vi "Wind_Turbine.vi"() -> (5 "Plug in titles":string[](array[string]), 7 "Plug in values":string[](array[string]))   [LabVIEW 2010]
uses:
  Globals/Meas_global.vi
  Globals/Plug_in_data_global.vi
  Globals/LDA_meas_global_1.vi
  Plug in sub vis/Wind_Turbine_Global.vi
  <vilib>/Analysis/NI_AALBase.lvlib
  <vilib>/Analysis/NI_AALPro.lvlib
panel:
  out "Angle 3":dbl format="%#_3g"
  out "Angle 2":dbl format="%#_3g"
  out "Angle 1":dbl format="%#_3g"
  out "L Status Phase lock index":i32
  out "Laser Status Index":i32
  out "Waveform Graph 3":dbl[](graph)
  out "Laser Phase lock index":i32
  out "Laser Disp Index":i32
  out "Av Variance 3":dbl
  out "Av Variance 2":dbl
  out "Av Variance 1":dbl
  out "slope 3":dbl format="%#_3g"
  out "slope 2":dbl format="%#_3g"
  out "Variance Blade 3":dbl[](graph)
  out "Variance Blade 2":dbl[](graph)
  out "Mean Blade 3":dbl[](graph)
  out "Mean Blade 2":dbl[](graph)
  out "Variance Blade 1":dbl[](graph)
  out "Av Disp 3":dbl
  out "Av Disp 2":dbl
  out "Av Disp 1":dbl
  out "slope 1":dbl format="%#_3g"
  in  "End Cut Deg":dbl
  in  "Start Cut Deg":dbl
  out "Waveform Graph 2":i16[](graph)
  out "Mean Blade 1":dbl[](graph)
  out "Array":i32[](array[numeric])
  in  "Angular Step":dbl=0.1
  in  "Turbine to Phase Lock to":u16(ring) items=["RV (WT1)"]
  in  "Change Dem Voltages?":bool
  out "All WTs":dbl[][](array[numeric]) format="%#.2g"
  out "WT trace index":i32[](array[numeric])
  in  "precision":string
  in  "Add Phase data to results file":bool
  in  "Separation Character":string="\t"
  in  "Output Directory":path
  in  "Save Phase averaged Profiles":bool
  out "LDA Chs":i32[](array[numeric])
  out "WT Stalled?":bool
  out "Pulse No":i32
  out "Last index":i32
  out "subarray":bool[](array[boolean])
  out "Index":i32[](array[numeric])
  out "Pulses per Rev":i32
  out "Av samples per pulse":i32
  out "Threshold":dbl
  in  "Channel to Phase lock":i32[](listbox)
  out "Last Block No of Revs":i32
  out "Hub RPM":dbl
  out "Generator trace":cluster{dbl, dbl, dbl[]}(graph)
  out "Hot wire trace":cluster{dbl, dbl, dbl[][]}(graph)
  out "Number of Revs":i32
  # "Mean RPM      SD RPM           Max-Min"
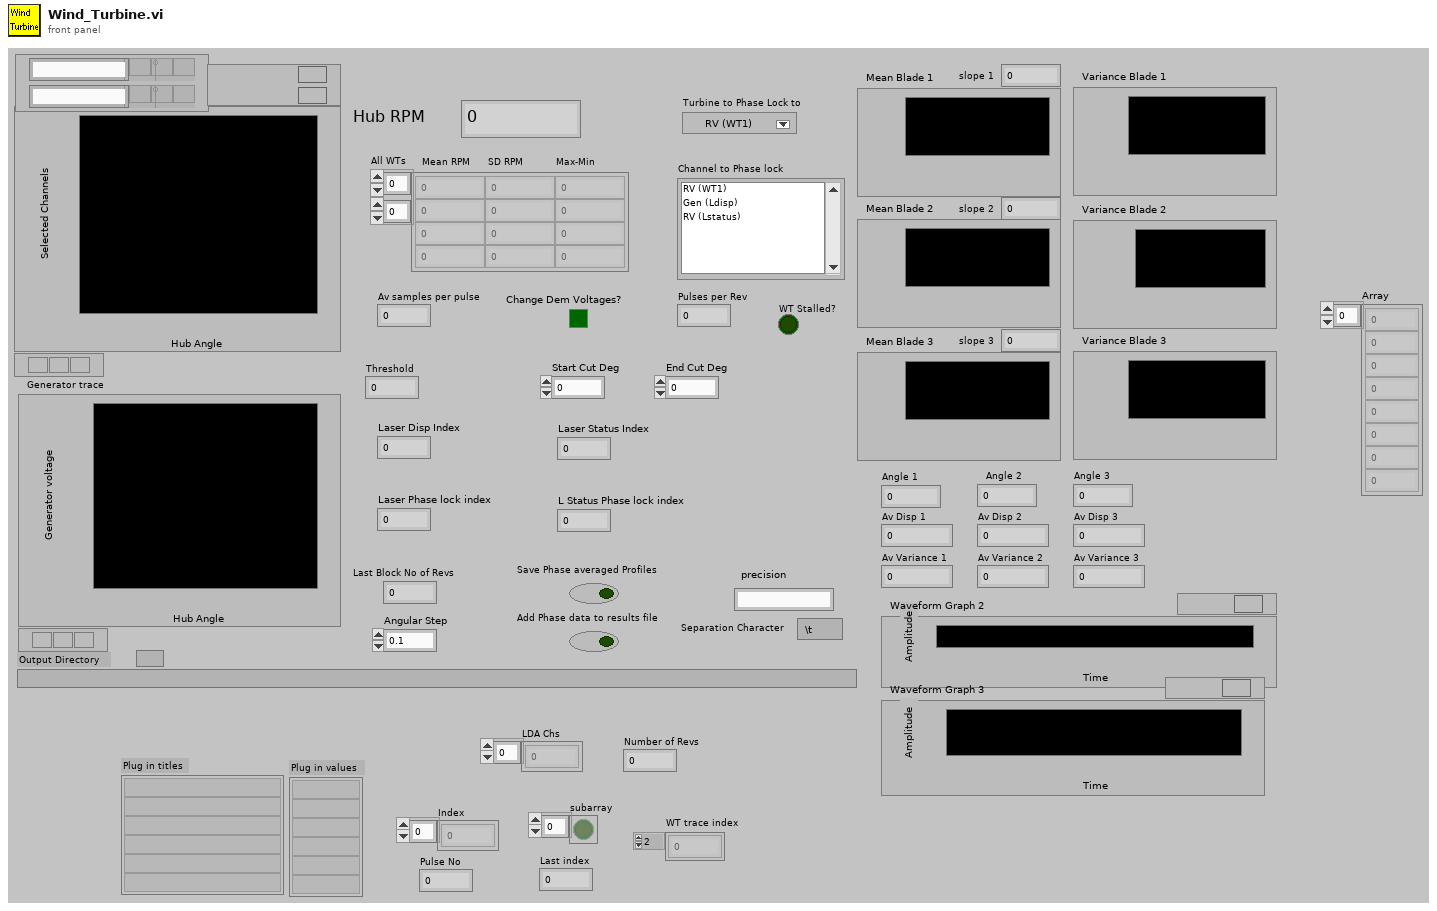
[diagram p1: front panel]
types:
  T1 = typedef "Analysis_info_cluster.ctl" = cluster{"Colour":u32, "Inst type":T2, "Inst name":string, "Symbol":string, "Code name":string, "Extra Info":string, "Inst Array":T3, "Index":i32, "Voltage Index":i32, "Extra Titles":string[], "Extra Values":string[]}
  T2 = typedef "Inst_type.ctl" = enum16{"Propeller anemometer", "Raw voltage", "Pressure Transducer", "Pitot-static tube", "Preston tube", "Hot wire", "Cross wire 1", "Cross wire 2", "Generic Linear", "Generic Polynomial", "Generic BackPoly", "Fast FID", "Thermocouple", "Cold wire", "Pulsed Wire", "LDA Vel", "LDA Tran time", "LDA Arr time"}
  T3 = typedef "Instrument_Array.ctl" = enum16{"PWA", "LDA", "Analogue"}
  T4 = typedef "Post_Process.ctl" = enum16{"Take New Data", "Post Process Raw Data File"}
  T5 = cluster{"Name":string, "X":dbl, "Y":dbl, "Z":dbl}[]
  T6 = cluster{"Name":string, "X":dbl, "Y":dbl, "Z":dbl}
  T7 = cluster{"[0]":bool, "[1]":bool, "[2]":bool, "[3]":bool}
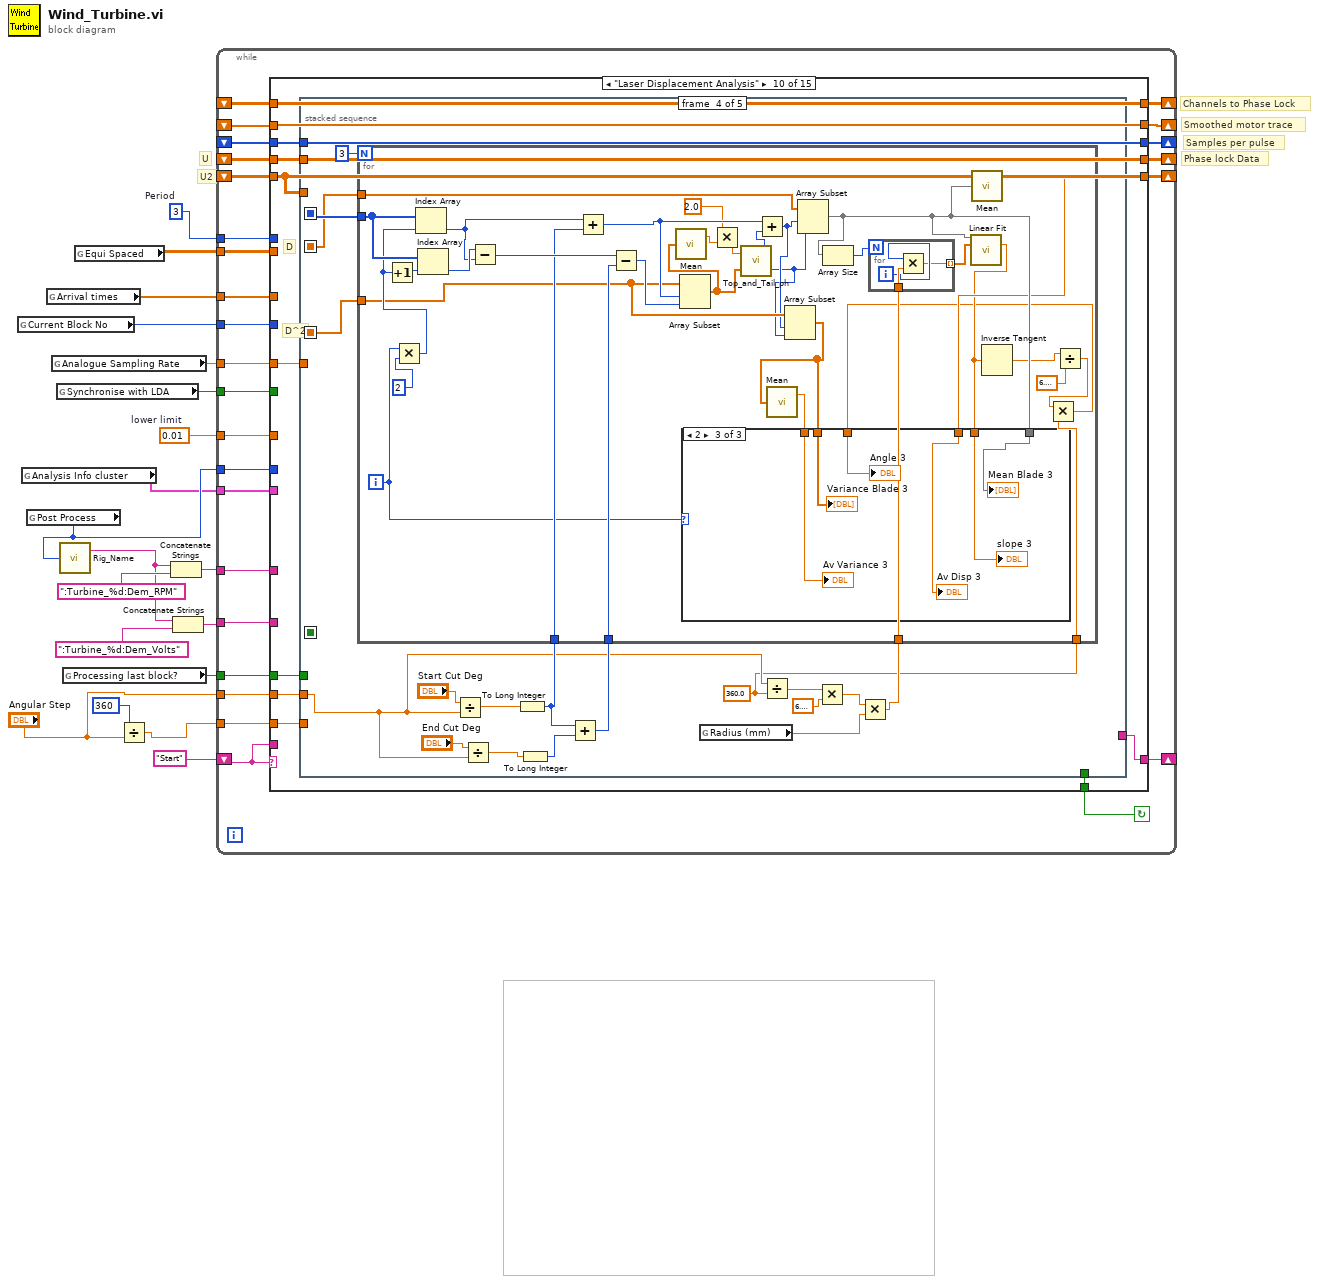
[diagram p0: block diagram]
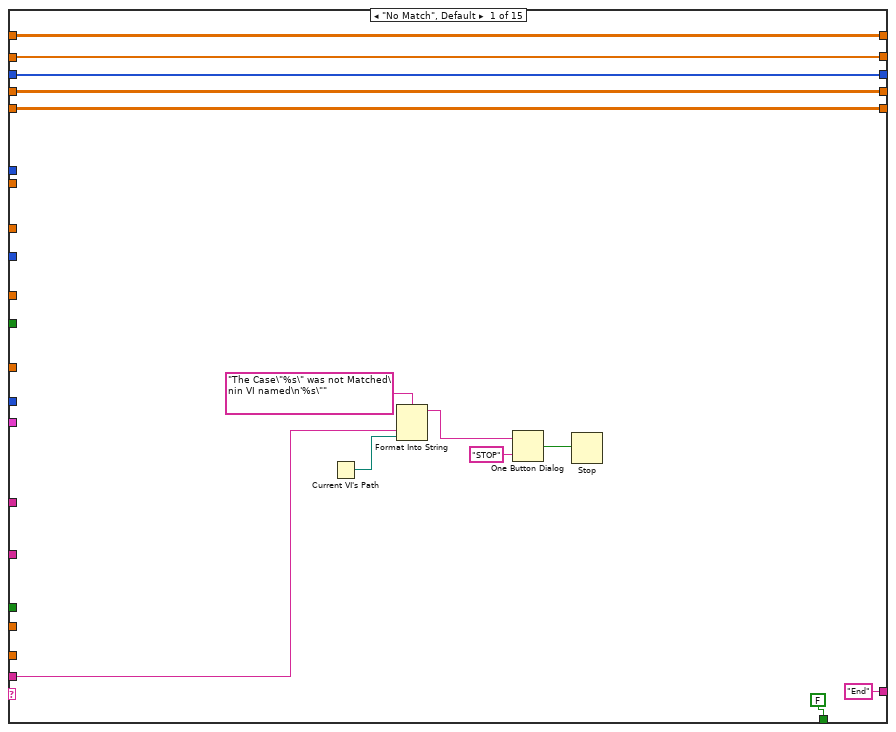
[diagram p2: hidden frame]
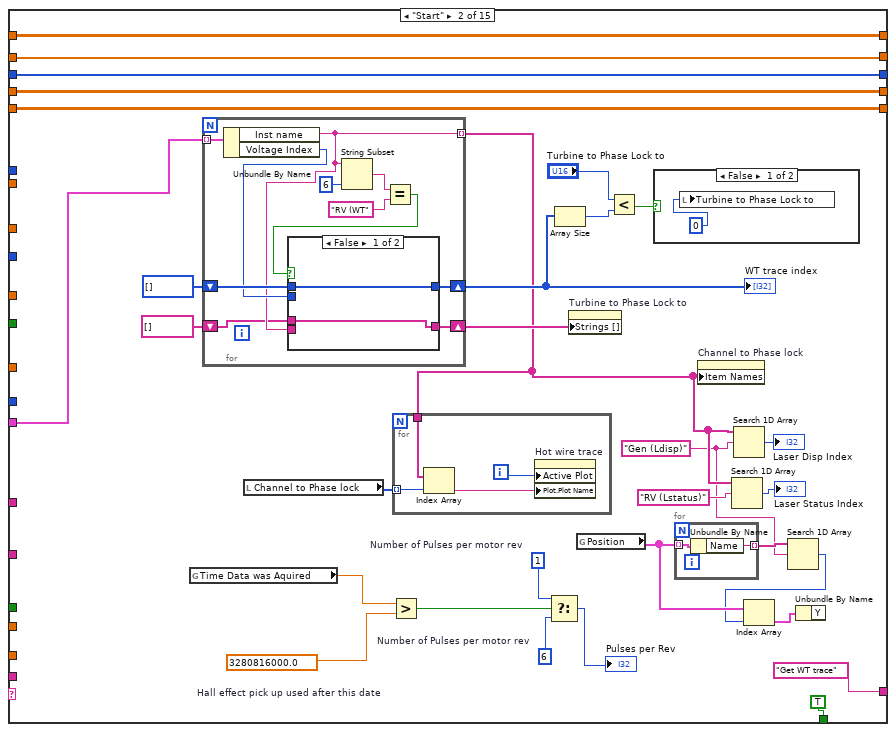
[diagram p3: hidden frame]
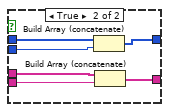
[diagram p5: hidden frame]
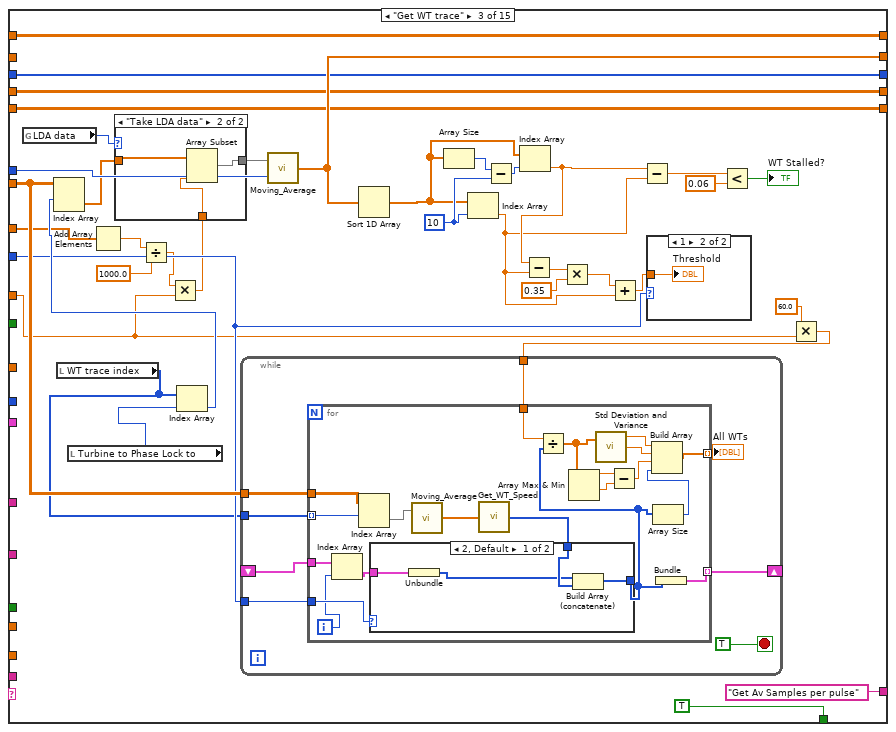
[diagram p6: hidden frame]
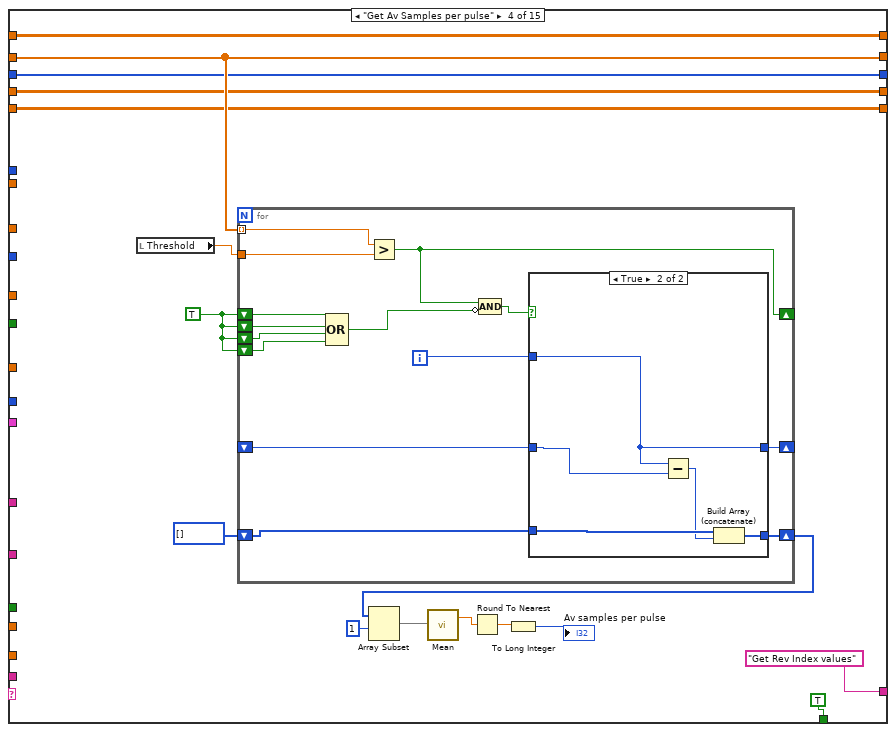
[diagram p10: hidden frame]
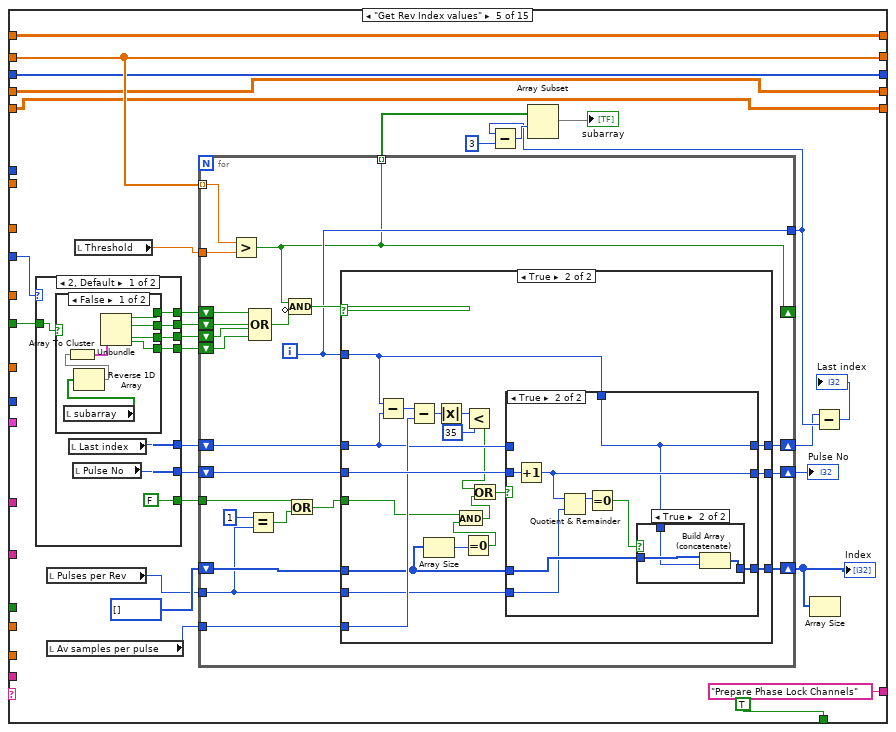
[diagram p12: hidden frame]
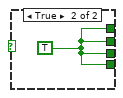
[diagram p13: hidden frame]
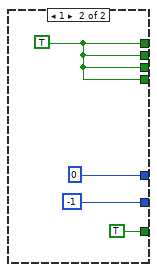
[diagram p14: hidden frame]
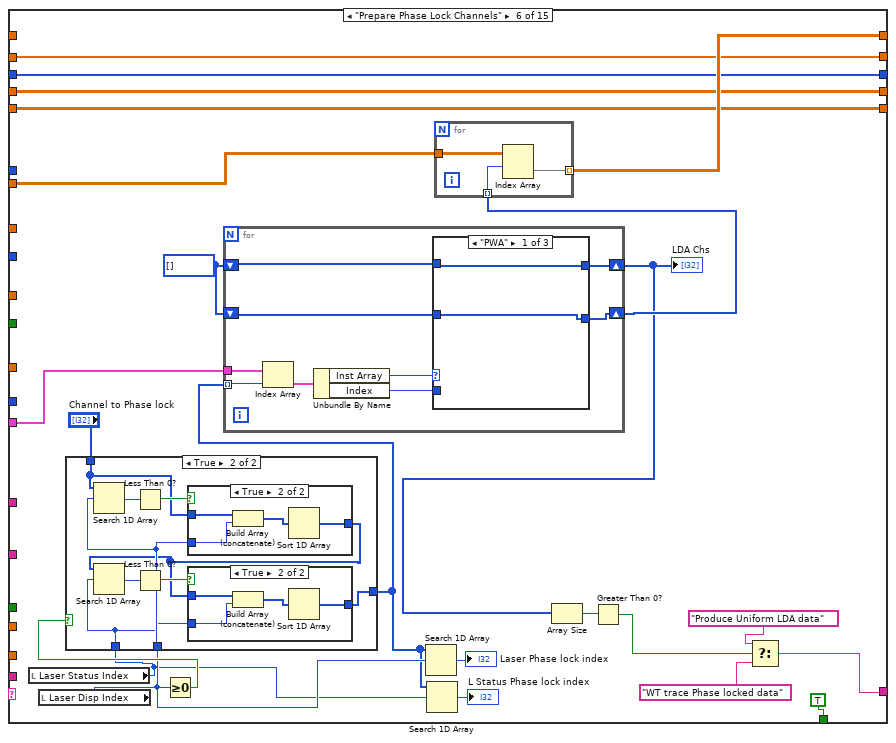
[diagram p18: hidden frame]
diagram:
  w16 = 3  # Period
  w17 = 0.01  # lower limit
  # "U"
  # "U2"
  # "Channels to Phase Lock"
  # "Phase lock Data"
  # "Samples per pulse"
  # "Smoothed motor trace"
  n1 = global read "Meas_global.vi" "Current Block No"() -> (w19:i32)
  n2 = global read "Meas_global.vi" "Analysis Info cluster"() -> (w8:T1[])
  n3 = global read "Meas_global.vi" "Post Process"() -> (w15:T4)
  n4 = global read "LDA_meas_global_1.vi" "Arrival times"() -> (w2:dbl[])
  n5 = global read "Meas_global.vi" "Analogue Sampling Rate"() -> (w18:dbl)
  n6 = global read "Meas_global.vi" "Synchronise with LDA"() -> (w9:bool)
  n7 = call "Rig_Name.vi"("Post Process"=w15) -> ("Rig Setup before dash"=w11:string)  [unwired: 1 out]
  n8 = global read "Meas_global.vi" "Processing last block?"() -> (w6:bool)
  n9 = global read "Plug_in_data_global.vi" "Equi Spaced"() -> (w5:dbl[][])
  n10 = Divide(x=360, y="Angular Step") -> (x/y=w3:dbl)
  n11 = Concatenate Strings(w11, ":Turbine_%d:Dem_RPM") -> (w10:string)
  n12 = Concatenate Strings(w11, ":Turbine_%d:Dem_Volts") -> (w14:string)
  n13 = while {
    tunnel: w19 -> [w46]
    tunnel: w5 -> [w45]
    shift-right: [w43] -> _
    shift-left: _ -> [w44]
    shift-right: [w42] -> _
    shift-left: _ -> [w41]
    tunnel: w18 -> [w40]
    tunnel: w14 -> [w39]
    tunnel: w10 -> [w38]
    tunnel: w17 -> [w37]
    tunnel: w16 -> [w36]
    tunnel: w15 -> [w35]
    tunnel: w9 -> [w34]
    tunnel: w8 -> [w33]
    shift-right: [w32] -> _
    shift-left: _ -> [w31]
    shift-right: [w30] -> _
    shift-left: "Start" -> [w28]
    tunnel: w6 -> [w27]
    shift-right: [w26] -> _
    shift-left: _ -> [w25]
    tunnel: w3 -> [w24]
    shift-right: [w22] -> _
    shift-left: _ -> [w23]
    tunnel: w2 -> [w21]
    tunnel: "Angular Step" -> [w20]
    stop <- w29 continue-if-true
    n14 = case shown="\"Laser Displacement Analysis\"" w28 {
      tunnel: w46 -> [_ _ w129 _ w256 _ _ w470 _ _ _ _ _ _ _]
      tunnel: w45 -> [_ _ w137 _ _ w356 w415 w466 _ _ _ _ _ _ _]
      tunnel: w44 -> [w51 w79 w141 w194 w234 w352 w423 w465 w526 w588 w770 w812 w839 w913 w927]
      tunnel: [w51 w79 w141 w194 w234 w352 w423 w464 w526 w588 w770 w812 w839 w913 w927] -> w43
      tunnel: [w52 w80 w142 w195 w235 w353 w424 w460 w527 w591 w768 w810 w847 w914 w932] -> w42
      tunnel: w41 -> [w52 w80 w142 w195 w235 w353 w424 w450 w527 w591 w768 w810 w847 w914 w932]
      tunnel: w40 -> [_ _ w124 _ _ _ w418 _ w537 w592 _ _ _ _ w931]
      tunnel: w39 -> [_ _ _ _ _ _ _ _ _ _ w775 w808 _ _ _]
      tunnel: w38 -> [_ _ _ _ _ _ _ _ _ _ w774 w783 _ _ _]
      tunnel: w37 -> [_ _ _ _ _ _ _ _ _ _ _ _ _ _ _]
      tunnel: w36 -> [_ _ w153 _ _ _ _ _ _ _ _ _ _ _ _]
      tunnel: w35 -> [_ _ _ _ _ _ _ _ _ _ w773 _ _ _ _]
      tunnel: w34 -> [_ _ _ _ w241 _ _ _ _ _ _ _ _ _ _]
      tunnel: w33 -> [_ w84 _ _ _ w359 _ _ _ _ _ _ _ _ _]
      tunnel: [w53 w81 w146 w196 w236 w354 w425 w459 w528 w590 w771 w813 w848 w915 w933] -> w32
      tunnel: w31 -> [w53 w81 _ w196 w236 w354 w425 w459 w528 w590 w771 w813 w848 w915 w933]
      tunnel: ["End" "Get WT trace" "Get Av Samples per pulse" "Get Rev Index values" "Prepare Phase Lock Channels" w348 "WT trace Phase locked data" ("f") "Output WT Statistics" w532 w582 w772 "End" ("f") "Check Folder Name" "Save Phase locked data" "End"] -> w30
      tunnel: [FALSE ("Change Control Voltage?") TRUE ("Processing last block?") TRUE TRUE ("Processing last block?") TRUE ("Change Control Voltage?") TRUE ("Change Control Voltage?") TRUE ("Change Control Voltage?") TRUE ("Change Control Voltage?") TRUE ("Change Control Voltage?") w583 w766 FALSE ("Change Control Voltage?") w844 w905 FALSE ("Change Control Voltage?")] -> w29
      tunnel: w28 -> [w54 _ _ _ _ _ _ _ _ _ _ _ _ _ _]
      tunnel: w27 -> [_ _ _ _ _ _ _ _ _ w584 w765 _ w842 _ _]
      tunnel: [w48 w78 w140 w193 w231 w355 w403 w454 w529 w589 w769 w811 w846 w912 w930] -> w26
      tunnel: w25 -> [w48 w78 w140 w193 w231 _ w406 w454 w529 w589 w769 w811 w846 w912 w930]
      tunnel: w24 -> [_ _ _ _ _ _ _ w453 _ w587 _ _ w840 _ w925]
      tunnel: w23 -> [w47 w76 w139 w192 w230 w344 w404 w447 w525 w585 w767 w809 w838 w903 w926]
      tunnel: [w47 w76 w139 w192 w230 w344 w404 w446 w525 w585 w767 w809 w838 w903 w926] -> w22
      tunnel: w21 -> [_ _ w127 _ _ _ w402 _ _ _ _ _ _ _ _]
      tunnel: w20 -> [_ _ _ _ _ _ _ _ w536 w586 _ _ _ _ _]
      frame "No Match", Default {
        n15 = Current VI's Path() -> (path=w55:path)
        n16 = Format Into String(format string="The Case\"%s\" was not Matched\nin VI named\n'%s\"" ("Format String"), w54, w55) -> (resulting string=w58:string)  [unwired: 2 in, 1 out]
        n17 = One Button Dialog(message=w58, button name ("OK")="STOP") -> (true=w56:bool)
        n18 = Stop(stop? (T)=w56) -> ()
      }
      frame "Start" {
        w63 = "Gen (Ldisp)"
        w85 = 6  # Number of Pulses per motor rev
        w86 = 1  # Number of Pulses per motor rev
        w88 = 3280816000.0  # Hall effect pick up used after this date
        n19 = global read "Meas_global.vi" "Time Data was Aquired"() -> (w89:dbl)
        n20 = for {
          tunnel: w84 -> [w108] mode=indexing
          tunnel: [w100] -> w66 mode=indexing
          shift-right: [w102] -> w71
          shift-left: i32[] [] -> [w103]
          shift-right: [w99] -> w73
          shift-left: string[] [] -> [w98]
          n21 = Unbundle By Name(w108) -> ("Inst name"=w100:string, "Voltage Index"=w101:i32)
          n22 = String Subset(string=w100, length (rest)=6 ("length (rest)")) -> (substring=w105:string)  [unwired: 1 out]
          n23 = Equal?(x=w105, y="RV (WT") -> (x = y?=w104:bool)
          n24 = case shown="False" w104 {
            tunnel: w103 -> [w110 w116]
            tunnel: [w110 w114] -> w102
            tunnel: w101 -> [_ w115]
            tunnel: w100 -> [_ w113]
            tunnel: [w109 w112] -> w99
            tunnel: w98 -> [w109 w111]
            frame False {
            }
            frame True {
              n25 = Build Array (concatenate)(w116, w115) -> (w114:i32[])
              n26 = Build Array (concatenate)(w111, w113) -> (w112:string[])
            }
          }
        }
        "WT trace index" <- w71
        n27 = local read "Channel to Phase lock"() -> (w77:i32[])
        n28 = Greater?(x=w89, y=w88) -> (0:w87:bool)
        n29 = for {
          tunnel: w66 -> [w97]
          tunnel: w77 -> [w96] mode=indexing
          i -> [w95]
          n30 = Index Array(array=w97, index=w96) -> (element=w94:string)
          n31 = property on="Hot wire trace" class="WFGraph (strict)"("Active Plot"=w95, "Plot.Plot Name"=w94) -> ()  [unwired: 2 in, 2 out]
        }
        n32 = Select(t=w86, s=w87, f=w85) -> (s? t:f=→"Pulses per Rev":i32)
        n33 = Array Size(array=w71) -> (size(s)=w72:i32)
        n34 = property on="Turbine to Phase Lock to" class="Ring (strict)"("Strings []"=w73) -> ()  [unwired: 2 in, 2 out]
        n35 = global read "Meas_global.vi" "Position"() -> (w62:T5)
        n36 = Less?(x="Turbine to Phase Lock to", y=w72) -> (x < y?=w69:bool)
        n37 = case shown="False" w69 {
          frame False {
            n38 = local write "Turbine to Phase Lock to"(0) -> ()
          }
          frame True {
          }
        }
        n39 = for {
          tunnel: w62 -> [w92] mode=indexing
          tunnel: [w91] -> w64 mode=indexing
          n40 = Unbundle By Name(w92) -> ("Name"=w91:string)
        }
        n41 = property on="Channel to Phase lock" class="LstBox (strict)"("Item Names"=w66) -> ()  [unwired: 2 in, 2 out]
        n42 = Search 1D Array(1D array=w66, element="RV (Lstatus)") -> (index of element=→"Laser Status Index":i32)  [unwired: 1 in]
        n43 = Search 1D Array(1D array=w66, element=w63) -> (index of element=→"Laser Disp Index":i32)  [unwired: 1 in]
        n44 = Search 1D Array(1D array=w64, element=w63) -> (index of element=w61:i32)  [unwired: 1 in]
        n45 = Index Array(array=w62, index=w61) -> (element=w60:T6)
        n46 = Unbundle By Name(w60) -> ()  [unwired: 1 out]
      }
      frame "Get WT trace" {
        w151 = 10 ("index")
        n47 = global read "Meas_global.vi" "LDA data"() -> (w119:enum16{"No LDA data", "Take LDA data"})
        n48 = local read "WT trace index"() -> (w118:i32[])
        n49 = local read "Turbine to Phase Lock to"() -> (w117:u16)
        n50 = Add Array Elements(numeric array=w127) -> (sum=w126:dbl)
        n51 = Divide(x=w126, y=1000.0) -> (x/y=w123:dbl)
        n52 = Multiply(x=w123, y=w124) -> (x*y=w120:dbl)
        n53 = Index Array(array=w118, index=w117) -> (element=w138:i32)
        n54 = Index Array(array=w137, index (row)=w138) -> (element=w122:dbl[])  [unwired: 1 in]
        n55 = case shown="\"Take LDA data\"" w119 {
          tunnel: w122 -> [w154 w157]
          tunnel: [w154 w156] -> w121
          tunnel: w120 -> [_ w155]
          frame "No LDA data" {
          }
          frame "Take LDA data" {
            n56 = Array Subset(array=w157, length=w155) -> (w156:dbl[])  [unwired: 1 in]
          }
        }
        n57 = call "Moving_Average.vi"("Period"=w153, "Input Array"=w121) -> ("N+1-Period"=w146:dbl[])
        n58 = Sort 1D Array(array=w146) -> (sorted array=w149:dbl[])
        n59 = Array Size(array=w149) -> (size(s)=w152:i32)
        n60 = Index Array(array=w149, index=w151) -> (element=w130:dbl)
        n61 = Subtract(x=w152, y=w151) -> (x-y=w150:i32)
        n62 = Index Array(array=w149, index=w150) -> (element=w131:dbl)
        n63 = Subtract(x=w131, y=w130) -> (x-y=w134:dbl)
        n64 = Multiply(x=w134, y=0.35) -> (x*y=w132:dbl)
        n65 = Add(x=w132, y=w130) -> (x+y=w128:dbl)
        n66 = Subtract(x=w131, y=w130) -> (x-y=w147:dbl)
        n67 = case shown="1" w129 {
          tunnel: w128 -> [_ w158]
          frame 0, Default {
          }
          frame 1 {
            "Threshold" <- w158
          }
        }
        n68 = Less?(x=w147, y=0.06) -> (x < y?=→"WT Stalled?":bool)
        n69 = Multiply(x=60.0, y=w124) -> (x*y=w135:dbl)
        n70 = while {
          tunnel: w118 -> [w166]
          tunnel: w137 -> [w165]
          tunnel: w129 -> [w164]
          shift-right: [w159] -> _
          shift-left: _ -> [w163]
          tunnel: w135 -> [w162]
          stop <- TRUE stop-if-true
          n71 = for {
            tunnel: w166 -> [w185] mode=indexing
            tunnel: w165 -> [w184]
            tunnel: w164 -> [w182]
            tunnel: w163 -> [w172]
            tunnel: w162 -> [w180]
            tunnel: [w173] -> w160 mode=indexing
            tunnel: [w167] -> w159 mode=indexing
            i -> [w171]
            n72 = Index Array(array=w172, index=w171) -> (element=w170:cluster{"Samples per pulse":i32[]})
            n73 = Index Array(array=w184, index (row)=w185) -> (element=w186:dbl[])  [unwired: 1 in]
            n74 = call "Moving_Average.vi"("Input Array"=w186) -> ("N+1-Period"=w183:dbl[])  [unwired: 1 in]
            n75 = call "Get_WT_Speed.vi"("Opto Trace"=w183) -> ("Samples per pulse"=w181:i32[])
            n76 = case shown="2, Default" w182 {
              tunnel: [w189 w191] -> w168
              tunnel: w181 -> [w190 w191]
              tunnel: w170 -> [w188 _]
              frame 2, Default {
                n77 = Unbundle(w188) -> ("Samples per pulse"=w187:i32[])
                n78 = Build Array (concatenate)(w187, w190) -> (w189:i32[])
              }
              frame 1 {
              }
            }
            n79 = Divide(x=w180, y=w168) -> (x/y=w177:dbl[])
            n80 = Array Max & Min(array=w177) -> (max value=w179:dbl, min value=w178:dbl)  [unwired: 2 out]
            n81 = call <vilib>:"Std Deviation and Variance.vi"("X"=w177) -> ("mean"=w176:dbl, "standard deviation"=w175:dbl)  [unwired: 1 in, 1 out]
            n82 = Subtract(x=w179, y=w178) -> (x-y=w174:dbl)
            n83 = Array Size(array=w168) -> (size(s)=w169:i32)
            n84 = Build Array(w176, w175, w174, w169) -> (w173:dbl[])
            n85 = Bundle("Samples per pulse"=w168) -> (w167:cluster{"Samples per pulse":i32[]})  [unwired: 1 in]
          }
          "All WTs" <- w160
        }
      }
      frame "Get Av Samples per pulse" {
        w205 = TRUE
        n86 = local read "Threshold"() -> (w199:dbl)
        n87 = for {
          shift-right: [w208] -> _
          shift-left: w205 -> [w213]
          shift-right: [w218] -> _
          shift-left: _ -> [w217]
          tunnel: w196 -> [w221] mode=indexing
          tunnel: w199 -> [w220]
          shift-right: [w215] -> w204
          shift-left: i32[] [] -> [w216]
          shift-left: w205 -> [w212]
          shift-left: w205 -> [w211]
          shift-left: w205 -> [w209]
          i -> [w214]
          n88 = Compound Arithmetic op=OR(w213, w212, w211, w209) -> (w210:bool)
          n89 = Greater?(x=w221, y=w220) -> (0:w208:bool)
          n90 = Compound Arithmetic op=AND(w208, invert w210) -> (w219:bool)
          n91 = case shown="True" w219 {
            tunnel: [w223 w226] -> w218
            tunnel: w214 -> [_ w226]
            tunnel: w217 -> [w223 w225]
            tunnel: w216 -> [w222 w228]
            tunnel: [w222 w227] -> w215
            frame False {
            }
            frame True {
              n92 = Subtract(x=w226, y=w225) -> (x-y=w224:i32)
              n93 = Build Array (concatenate)(w228, w224) -> (w227:i32[])
            }
          }
        }
        n94 = Array Subset(array=w204, index=1) -> (w202:i32[])  [unwired: 1 in]
        n95 = call <vilib>:"Mean.vi"("X"=w202) -> ("mean"=w201:dbl)  [unwired: 1 out]
        n96 = Round To Nearest(number=w201) -> (nearest integer value=w200:dbl)
        n97 = To Long Integer(number=w200) -> (32bit integer=→"Av samples per pulse":i32)
      }
      frame "Get Rev Index values" {
        n98 = case shown="2, Default" w256 {
          tunnel: [w258 -1] -> w255
          tunnel: [w259 0] -> w253
          tunnel: [w265 w274] -> w248
          tunnel: [w264 w274] -> w247
          tunnel: [w263 w274] -> w246
          tunnel: [w262 w274] -> w245
          tunnel: [FALSE TRUE] -> w244
          tunnel: w241 -> [w260 _]
          frame 2, Default {
            n99 = case shown="False" w260 {
              tunnel: [w270 w273] -> w265
              tunnel: [w269 w273] -> w264
              tunnel: [w268 w273] -> w263
              tunnel: [w267 w273] -> w262
              frame False {
                n100 = local read "subarray"() -> (w266:bool[])
                n101 = Reverse 1D Array(array=w266) -> (reversed array=w272:bool[])
                n102 = Array To Cluster(array=w272) -> (cluster=w271:T7)
                n103 = Unbundle(w271) -> ("[0]"=w270:bool, "[1]"=w269:bool, "[2]"=w268:bool, "[3]"=w267:bool)
              }
              frame True {
                w273 = TRUE ("[0]")
              }
            }
            n104 = local read "Last index"() -> (w259:i32)
            n105 = local read "Pulse No"() -> (w258:i32)
          }
          frame 1 {
            w274 = TRUE
          }
        }
        n106 = local read "Pulses per Rev"() -> (w238:i32)
        n107 = local read "Av samples per pulse"() -> (w239:i32)
        n108 = local read "Threshold"() -> (w240:dbl)
        n109 = for {
          shift-right: [w285] -> _
          shift-left: w248 -> [w289]
          shift-right: [w296] -> w242
          shift-left: w253 -> [w293]
          tunnel: w236 -> [w299] mode=indexing
          tunnel: w240 -> [w298]
          shift-right: [w294] -> w237
          shift-left: w255 -> [w295]
          shift-right: [w291] -> w229
          shift-left: i32[] [] -> [w292]
          tunnel: [w290] -> w243
          shift-left: w247 -> [w288]
          shift-left: w246 -> [w287]
          tunnel: [w285] -> w250 mode=indexing
          shift-left: w245 -> [w284]
          tunnel: w239 -> [w283]
          tunnel: w244 -> [w279]
          tunnel: w238 -> [w282]
          i -> [w290]
          n110 = Greater?(x=w299, y=w298) -> (0:w285:bool)
          n111 = Equal?(x=1, y=w282) -> (x = y?=w280:bool)
          n112 = Compound Arithmetic op=OR(w289, w288, w287, w284) -> (w286:bool)
          n113 = Or(x=w279, y=w280) -> (x .or. y?=w278:bool)
          n114 = Compound Arithmetic op=AND(w285, invert w286) -> (w297:bool)
          n115 = case shown="True" w297 {
            tunnel: [w302 w312] -> w296
            tunnel: w290 -> [_ w318]
            tunnel: w295 -> [w301 w321]
            tunnel: [w301 w320] -> w294
            tunnel: w293 -> [w302 w311]
            tunnel: w292 -> [w300 w310]
            tunnel: [w300 w319] -> w291
            tunnel: w283 -> [_ w316]
            tunnel: w278 -> [_ w305]
            tunnel: w282 -> [_ w304]
            frame False {
            }
            frame True {
              n116 = Subtract(x=w318, y=w311) -> (x-y=w317:i32)
              n117 = Subtract(x=w317, y=w316) -> (x-y=w315:i32)
              n118 = Array Size(array=w310) -> (size(s)=w308:i32)
              n119 = Absolute Value(x=w315) -> (abs(x)=w314:i32)
              n120 = Equal To 0?(x=w308) -> (x = 0?=w307:bool)
              n121 = And(x=w305, y=w307) -> (x .and. y?=w306:bool)
              n122 = Less?(x=w314, y=35) -> (x < y?=w303:bool)
              n123 = Or(x=w303, y=w306) -> (x .or. y?=w309:bool)
              n124 = case shown="True" w309 {
                tunnel: w321 -> [w324 w332]
                tunnel: [w324 w331] -> w320
                tunnel: w310 -> [w323 w328]
                tunnel: [w323 w327] -> w319
                tunnel: w318 -> [_ w326]
                tunnel: [w322 w326] -> w312
                tunnel: w311 -> [w322 _]
                tunnel: w304 -> [_ w325]
                frame False {
                }
                frame True {
                  n125 = Increment(x=w332) -> (x+1=w331:i32)
                  n126 = Quotient & Remainder(x=w331, y=w325) -> (x-y*floor(x/y)=w330:i32)  [unwired: 1 out]
                  n127 = Equal To 0?(x=w330) -> (x = 0?=w329:bool)
                  n128 = case shown="True" w329 {
                    tunnel: w328 -> [w333 w336]
                    tunnel: w326 -> [_ w335]
                    tunnel: [w333 w334] -> w327
                    frame False {
                    }
                    frame True {
                      n129 = Build Array (concatenate)(w336, w335) -> (w334:i32[])
                    }
                  }
                }
              }
            }
          }
        }
        "Index" <- w229
        "Pulse No" <- w237
        n130 = Subtract(x=w243, y=3) -> (x-y=w251:i32)
        n131 = Array Subset(array=w250, index=w251) -> (→"subarray":bool[])  [unwired: 1 in]
        n132 = Array Size(array=w229) -> ()  [unwired: 1 out]
        n133 = Subtract(x=w242, y=w243) -> (x-y=→"Last index":i32)
      }
      frame "Prepare Phase Lock Channels" {
        w358 = i32[] []
        n134 = local read "Laser Status Index"() -> (w337:i32)
        n135 = local read "Laser Disp Index"() -> (w341:i32)
        n136 = Greater Or Equal To 0?(x=w341) -> (x >= 0?=w343:bool)
        n137 = case shown="True" w343 {
          tunnel: "Channel to Phase lock" -> [w360 w367]
          tunnel: w341 -> [_ w366]
          tunnel: [w360 w363] -> w338
          tunnel: w337 -> [_ w361]
          frame False {
          }
          frame True {
            n138 = Search 1D Array(1D array=w367, element=w366) -> (index of element=w369:i32)  [unwired: 1 in]
            n139 = Less Than 0?(x=w369) -> (x < 0?=w368:bool)
            n140 = case shown="True" w368 {
              tunnel: w367 -> [w375 w379]
              tunnel: w366 -> [_ w378]
              tunnel: [w375 w376] -> w362
              frame False {
              }
              frame True {
                n141 = Build Array (concatenate)(w379, w378) -> (w377:i32[])
                n142 = Sort 1D Array(array=w377) -> (sorted array=w376:i32[])
              }
            }
            n143 = Search 1D Array(1D array=w362, element=w361) -> (index of element=w364:i32)  [unwired: 1 in]
            n144 = Less Than 0?(x=w364) -> (x < 0?=w365:bool)
            n145 = case shown="True" w365 {
              tunnel: w362 -> [w370 w374]
              tunnel: w361 -> [_ w373]
              tunnel: [w370 w371] -> w363
              frame False {
              }
              frame True {
                n146 = Build Array (concatenate)(w374, w373) -> (w372:i32[])
                n147 = Sort 1D Array(array=w372) -> (sorted array=w371:i32[])
              }
            }
          }
        }
        n148 = for {
          tunnel: w338 -> [w391] mode=indexing
          tunnel: w359 -> [w390]
          shift-right: [w383] -> w357
          shift-left: w358 -> [w384]
          shift-right: [w385] -> w350
          shift-left: w358 -> [w386]
          n149 = Index Array(array=w390, index=w391) -> (element=w389:T1)
          n150 = Unbundle By Name(w389) -> ("Inst Array"=w388:T3, "Index"=w387:i32)
          n151 = case shown="\"PWA\"" w388 {
            tunnel: w387 -> [_ w397 w401]
            tunnel: w386 -> [w393 w396 w398]
            tunnel: [w393 w395 w398] -> w385
            tunnel: w384 -> [w392 w394 w400]
            tunnel: [w392 w394 w399] -> w383
            frame "PWA" {
            }
            frame "LDA" {
              n152 = Build Array (concatenate)(w396, w397) -> (w395:i32[])
            }
            frame "Analogue" {
              n153 = Build Array (concatenate)(w400, w401) -> (w399:i32[])
            }
          }
        }
        "LDA Chs" <- w350
        n154 = Search 1D Array(1D array=w338, element=w341) -> (index of element=→"Laser Phase lock index":i32)  [unwired: 1 in]
        n155 = Search 1D Array(1D array=w338, element=w337) -> (index of element=→"L Status Phase lock index":i32)  [unwired: 1 in]
        n156 = for {
          tunnel: w357 -> [w382] mode=indexing
          tunnel: w356 -> [w381]
          tunnel: [w380] -> w355 mode=indexing
          n157 = Index Array(array=w381, index (row)=w382) -> (element=w380:dbl[])  [unwired: 1 in]
        }
        n158 = Array Size(array=w350) -> (size(s)=w351:i32)
        n159 = Greater Than 0?(x=w351) -> (x > 0?=w349:bool)
        n160 = Select(t="Produce Uniform LDA data", s=w349, f="WT trace Phase locked data") -> (s? t:f=w348:string)
      }
      frame "Produce Uniform LDA data" {
        n161 = Reciprocal(x=w418) -> (1/x=w419:dbl)
        n162 = Multiply(x=w419, y=1000.0) -> (x*y=w416:dbl)
        n163 = for {
          shift-right: [w437] -> _
          shift-left: 0.0 -> [w439]
          tunnel: w402 -> [w438] mode=indexing
          tunnel: [w437] -> w405 mode=indexing
          n164 = Add(x=w439, y=w438) -> (x+y=w437:dbl)
        }
        n165 = Array Size(array=w415) -> (size(s)=w414:i32[])
        n166 = Index Array(array=w414, index=1) -> (element=w412:i32)
        n167 = global read "Plug_in_data_global.vi" "Vari Spaced"() -> (w409:dbl[][])
        n168 = for {
          N: w412 -> [_]
          tunnel: w416 -> [w435]
          tunnel: w405 -> [w434]
          tunnel: [w433] -> w411 mode=indexing
          i -> [w436]
          n169 = Multiply(x=w435, y=w436) -> (x*y=w432:dbl)
          n170 = Threshold 1D Array(2:w432, 3:w434) -> (0:w433:dbl)  [unwired: 1 out]
        }
        n171 = local read "LDA Chs"() -> (w410:i32[])
        n172 = for {
          tunnel: w410 -> [w442] mode=indexing
          tunnel: w409 -> [w441]
          tunnel: [w440] -> w408 mode=indexing
          n173 = Index Array(array=w441, index (row)=w442) -> (element=w440:dbl[])  [unwired: 1 in]
        }
        n174 = for {
          tunnel: [w428] -> w407 mode=indexing
          tunnel: w408 -> [w427] mode=indexing
          tunnel: w411 -> [w426]
          n175 = for {
            tunnel: [w431] -> w428 mode=indexing
            tunnel: w427 -> [w430]
            tunnel: w426 -> [w429] mode=indexing
            n176 = Interpolate 1D Array(1:w429, 2:w430) -> (0:w431:dbl)
          }
        }
        n177 = Build Array (concatenate)(w407, w406) -> (w403:dbl[][])
      }
      frame "WT trace Phase locked data" {
        n178 = local read "Index"() -> (w462:i32[])
        n179 = local read "Turbine to Phase Lock to"() -> (w443:u16)
        n180 = local read "WT trace index"() -> (w445:i32[])
        n181 = local read "Number of Revs"() -> (w463:i32)
        n182 = Array Subset(array=w462, index=1) -> (w469:i32[])  [unwired: 1 in]
        n183 = Index Array(array=w462, index=0) -> (element=w468:i32)
        n184 = Index Array(array=w445, index=w443) -> (element=w444:i32)
        n185 = Index Array(array=w466, index (row)=w444) -> (element=w456:dbl[])  [unwired: 1 in]
        n186 = Array Size(array=w469) -> (size(s)=w448:i32)
        "Last Block No of Revs" <- w448
        n187 = case shown="2, Default" w470 {
          tunnel: [w475 w480] -> w461
          tunnel: w448 -> [w476 w480]
          tunnel: w463 -> [w477 _]
          tunnel: [FALSE TRUE] -> w467
          tunnel: [w473 i32[] []] -> w451
          tunnel: w450 -> [w473 _]
          frame 2, Default {
            n188 = Add(x=w477, y=w476) -> (x+y=w475:i32)
          }
          frame 1 {
          }
        }
        "Number of Revs" <- w461
        n189 = Build Array (concatenate)(w456, w454) -> (w455:dbl[][])
        n190 = Increment(x=w453) -> (x+1=w452:dbl)
        n191 = for {
          shift-right: [w496] -> _
          shift-left: w468 -> [w489]
          tunnel: w469 -> [w496] mode=indexing
          tunnel: w467 -> [w493]
          shift-right: [w491] -> w464
          shift-left: w465 -> [w490]
          tunnel: w455 -> [w492]
          tunnel: w452 -> [w487]
          tunnel: w453 -> [w486]
          tunnel: [w483] -> w449 mode=indexing
          shift-right: [w481] -> w446
          shift-left: w447 -> [w482]
          i -> [w495]
          n192 = Subtract(x=w496, y=w489) -> (x-y=w483:i32)
          n193 = Equal To 0?(x=w495) -> (x = 0?=w494:bool)
          n194 = Divide(x=w483, y=w486) -> (x/y=w488:dbl)
          n195 = for {
            N: w487 -> [_]
            tunnel: w489 -> [w501]
            tunnel: w488 -> [w499]
            tunnel: [w497] -> w485 mode=indexing
            i -> [w500]
            n196 = Multiply(x=w499, y=w500) -> (x*y=w498:dbl)
            n197 = Add(x=w501, y=w498) -> (x+y=w497:dbl)
          }
          n198 = And(x=w493, y=w494) -> (x .and. y?=w484:bool)
          n199 = for {
            tunnel: w492 -> [w510] mode=indexing
            tunnel: w484 -> [w513]
            tunnel: [w512] -> w491 mode=indexing
            tunnel: w490 -> [w508]
            tunnel: w485 -> [w509]
            tunnel: w482 -> [w507]
            tunnel: [w504] -> w481 mode=indexing
            i -> [w506]
            # "u^2"
            # "U"
            n200 = for {
              tunnel: w510 -> [w516]
              tunnel: [w515] -> w505 mode=indexing
              tunnel: w509 -> [w514] mode=indexing
              n201 = Interpolate 1D Array(1:w514, 2:w516) -> (0:w515:dbl)
            }
            n202 = Index Array(array=w508, index (row)=w506) -> (element=w511:dbl[])  [unwired: 1 in]
            n203 = Index Array(array=w507, index (row)=w506) -> (element=w502:dbl[])  [unwired: 1 in]
            n204 = Multiply(x=w505, y=w505) -> (x*y=w503:dbl[])
            n205 = case shown="False" w513 {
              tunnel: [w522 w524] -> w512
              tunnel: w505 -> [w520 w524]
              tunnel: w511 -> [w521 _]
              tunnel: [w518 w523] -> w504
              tunnel: w503 -> [w519 w523]
              tunnel: w502 -> [w517 _]
              frame False {
                n206 = Add(x=w521, y=w520) -> (x+y=w522:dbl[])
                n207 = Add(x=w517, y=w519) -> (x+y=w518:dbl[])
              }
              frame True {
              }
            }
          }
        }
        n208 = Build Array (concatenate)(w451, w449) -> (w460:i32[])
      }
      frame "Output WT Statistics" {
        w541 = string[] []
        n209 = Multiply(x=60.0, y=w537) -> (x*y=w556:dbl)
        n210 = Divide(x=w556, y=w527) -> (x/y=w555:dbl[])
        n211 = call <vilib>:"Std Deviation and Variance.vi"("X"=w555) -> ("mean"=→"Hub RPM":dbl)  [unwired: 1 in, 2 out]
        n212 = local read "All WTs"() -> (w543:dbl[][])
        n213 = local read "Number of Revs"() -> (w544:i32)
        n214 = for {
          tunnel: w543 -> [w569] mode=indexing
          shift-right: [w563] -> w542
          shift-left: w541 -> [w564]
          shift-right: [w559] -> w539
          shift-left: w541 -> [w561]
          tunnel: string[] ["WT_%d:Hub_RPM:Mean", "WT_%d:Hub_RPM:St_Dev", "WT_%d:Hub_RPM:Max-Min", "WT_%d:Number_of:Revs"] ("Plug in titles") -> [w562]
          i -> [w558]
          n215 = Index Array(array=w569, index=0) -> (element=w568:dbl)
          n216 = Index Array(array=w569, index=1) -> (element=w567:dbl)
          n217 = Index Array(array=w569, index=2) -> (element=w566:dbl)
          n218 = Index Array(array=w569, index=3) -> (element=w565:dbl)
          n219 = for {
            tunnel: w562 -> [w581] mode=indexing
            tunnel: [w579] -> w560 mode=indexing
            tunnel: w558 -> [w578]
            n220 = Increment(x=w578) -> (x+1=w580:i32)
            n221 = Format Into String(format string=w581, w580) -> (resulting string=w579:string)  [unwired: 2 in, 1 out]
          }
          n222 = call "Number_2_string.vi"("number"=w568) -> ("String"=w576:string)  [unwired: 1 in]
          n223 = call "Number_2_string.vi"("number"=w567) -> ("String"=w577:string)  [unwired: 1 in]
          n224 = call "Number_2_string.vi"("number"=w566) -> ("String"=w575:string)  [unwired: 1 in]
          n225 = Number To Decimal String(number=w565) -> (decimal integer string=w574:string)  [unwired: 1 out]
          n226 = Build Array (concatenate)(w564, w576, w577, w575, w574) -> (w563:string[])
          n227 = Build Array (concatenate)(w561, w560) -> (w559:string[])
        }
        "Plug in titles" <- w539
        "Plug in values" <- w542
        n228 = Index Array(array=w526, index (row)=0 ("index")) -> (element=w552:dbl[])  [unwired: 1 in]
        n229 = Array Subset(array=w526, index (row)=1 ("index")) -> (w550:dbl[][])  [unwired: 3 in]
        n230 = Divide(x=w550, y=w544) -> (x/y=w538:dbl[][])
        n231 = local read "Laser Disp Index"() -> (w534:i32)
        n232 = Divide(x=w552, y=w544) -> (x/y=w546:dbl[])
        n233 = Bundle(0.0, "Angular Step"=w536, w538) -> (→"Hot wire trace":cluster{dbl, "Angular Step":dbl, dbl[][]})  [unwired: 1 out]
        n234 = Bundle(0.0, "Angular Step"=w536, w546) -> (→"Generator trace":cluster{dbl, "Angular Step":dbl, dbl[]})  [unwired: 1 out]
        n235 = Greater Or Equal To 0?(x=w534) -> (x >= 0?=w533:bool)
        n236 = Select(t="Laser Displacement Analysis", s=w533, f="Get Last Block info") -> (s? t:f=w532:string)
      }
      frame "Laser Displacement Analysis" {
        # "D^2"
        # "D"
        n237 = stacked-sequence {
          seq-local: [_ w609 _ _ _] -> [_ _ w623 _ _]
          seq-local: [_ _ w624 _ _] -> [_ _ _ w664 _]
          seq-local: [w599 _ _ _ _] -> [_ _ _ w660 _]
          seq-local: [w596 _ _ _ _] -> [_ _ _ w659 _]
          tunnel: w592 -> [_ _ _ _ _]
          tunnel: w591 -> [_ _ _ _ _]
          tunnel: w588 -> [w606 w614 _ _ _]
          tunnel: w587 -> [_ _ _ _ _]
          tunnel: w586 -> [_ _ _ w658 _]
          tunnel: w585 -> [w607 _ _ _ _]
          tunnel: w584 -> [_ _ _ _ w727]
          tunnel: [_ _ _ _ TRUE] -> w583
          tunnel: [_ _ _ _ "Get Last Block info"] -> w582
          frame #0 {
            n238 = local read "Laser Phase lock index"() -> (w598:i32)
            n239 = local read "Number of Revs"() -> (w602:i32)
            n240 = Increment(x=w598) -> (x+1=w595:i32)
            n241 = Index Array(array=w607, index (row)=w595) -> (element=w604:dbl[])  [unwired: 1 in]
            n242 = Index Array(array=w606, index (row)=w595) -> (element=w603:dbl[])  [unwired: 1 in]
            n243 = Divide(x=w604, y=w602) -> (x/y=w593:dbl[])
            n244 = Divide(x=w603, y=w602) -> (x/y=w594:dbl[])
            "Waveform Graph 3" <- w594
            n245 = Build Array (concatenate)(w594, w594, 0.0) -> (w596:dbl[])
            n246 = Square(x=w594) -> (x^2=w605:dbl[])
            n247 = Subtract(x=w593, y=w605) -> (x-y=w601:dbl[])
            n248 = Build Array (concatenate)(w601, w601, 0.0) -> (w599:dbl[])
          }
          frame #1 {
            n249 = local read "L Status Phase lock index"() -> (w615:i32)
            n250 = local read "Number of Revs"() -> (w617:i32)
            n251 = Increment(x=w615) -> (x+1=w616:i32)
            n252 = Index Array(array=w614, index (row)=w616) -> (element=w618:dbl[])  [unwired: 1 in]
            n253 = Divide(x=w618, y=w617) -> (x/y=w612:dbl[])
            n254 = Build Array (concatenate)(w612, w612, 0.0) -> (w611:dbl[])
            n255 = Greater?(x=w611, y=0.4) -> (0:w609:bool[])
            n256 = Array Size(array=w609) -> (size(s)=w608:i32)
            n257 = Divide(x=w608, y=2) -> (x/y=w621:dbl)
            n258 = Boolean To (0,1)(Boolean=w609) -> (0, 1=w622:i16[])
            n259 = Array Subset(array=w622, length=w621) -> (→"Waveform Graph 2":i16[])  [unwired: 1 in]
          }
          frame #2 {
            n260 = Index Array(array=w623, index=0) -> (element=w626:bool)
            n261 = for {
              tunnel: w623 -> [w633] mode=indexing
              shift-right: [w633] -> _
              shift-left: w626 -> [w628]
              shift-right: [w630] -> w624
              shift-left: i32[] [] -> [w631]
              i -> [w632]
              n262 = Not Equal?(x=w633, y=w628) -> (x != y?=w629:bool)
              n263 = case shown="True" w629 {
                tunnel: w632 -> [_ w640]
                tunnel: w631 -> [w634 w638]
                tunnel: [w634 w639] -> w630
                tunnel: w628 -> [_ w635]
                frame False {
                }
                frame True {
                  n264 = Array Size(array=w638) -> (size(s)=w637:i32)
                  n265 = Equal To 0?(x=w637) -> (x = 0?=w636:bool)
                  n266 = case shown="False" w636 {
                    tunnel: w640 -> [w641 w647]
                    tunnel: w638 -> [w643 w646]
                    tunnel: [w642 w645] -> w639
                    tunnel: w635 -> [_ w644]
                    frame False {
                      n267 = Build Array (concatenate)(w643, w641) -> (w642:i32[])
                    }
                    frame True {
                      n268 = case shown="False" w644 {
                        tunnel: w647 -> [_ w651]
                        tunnel: w646 -> [w648 w650]
                        tunnel: [w648 w649] -> w645
                        frame False {
                        }
                        frame True {
                          n269 = Build Array (concatenate)(w650, w651) -> (w649:i32[])
                        }
                      }
                    }
                  }
                }
              }
            }
            "Array" <- w624
          }
          frame #3 {
            w653 = 360.0 ("y")
            n270 = Divide(x="Start Cut Deg", y=w658) -> (x/y=w666:dbl)
            n271 = Divide(x="End Cut Deg", y=w658) -> (x/y=w667:dbl)
            n272 = To Long Integer(number=w666) -> (32bit integer=w662:i32)
            n273 = To Long Integer(number=w667) -> (32bit integer=w665:i32)
            n274 = Add(x=w662, y=w665) -> (x+y=w661:i32)
            n275 = global read "Wind_Turbine_Global.vi" "Radius (mm)"() -> (w652:dbl)
            n276 = Divide(x=w658, y=w653) -> (x/y=w657:dbl)
            n277 = Multiply(x=w657, y=6.283185307179586) -> (x*y=w656:dbl)
            n278 = Multiply(x=w656, y=w652) -> (x*y=w654:dbl)
            n279 = for {
              N: 3 -> [_]
              tunnel: w659 -> [w700]
              tunnel: w664 -> [w697]
              tunnel: w662 -> [w693]
              tunnel: w661 -> [w692]
              tunnel: w654 -> [w691]
              tunnel: w660 -> [w682]
              tunnel: w653 -> [w675]
              i -> [w690]
              n280 = Multiply(x=w690, y=2) -> (x*y=w695:i32)
              n281 = Increment(x=w695) -> (x+1=w694:i32)
              n282 = Index Array(array=w697, index=w695) -> (element=w702:i32)
              n283 = Index Array(array=w697, index=w694) -> (element=w703:i32)
              n284 = Subtract(x=w703, y=w702) -> (x-y=w701:i32)
              n285 = Add(x=w702, y=w693) -> (x+y=w685:i32)
              n286 = Subtract(x=w701, y=w692) -> (x-y=w687:i32)
              n287 = Array Subset(array=w682, index=w685, length=w687) -> (w673:dbl[])
              n288 = call <vilib>:"Mean.vi"("X"=w673) -> ("mean"=w672:dbl)  [unwired: 1 out]
              n289 = Multiply(x=2.0, y=w672) -> (x*y=w670:dbl)
              n290 = call "Top_and_Tail_ph.vi"("Array in"=w673, "Threshold"=w670) -> ("Length"=w680:i32, "Start Index"=w684:i32)
              n291 = Add(x=w685, y=w684) -> (x+y=w681:i32)
              n292 = Array Subset(array=w682, index=w681, length=w680) -> (w683:dbl[])
              n293 = call <vilib>:"Mean.vi"("X"=w683) -> ("mean"=w686:dbl)  [unwired: 1 out]
              n294 = Array Subset(array=w700, index=w681, length=w680) -> (w689:dbl[])
              n295 = Array Size(array=w689) -> (size(s)=w699:i32)
              n296 = for {
                N: w699 -> [_]
                tunnel: w691 -> [w724]
                tunnel: [w722] -> w698 mode=indexing
                i -> [w723]
                n297 = Multiply(x=w723, y=w724) -> (x*y=w722:dbl)
              }
              n298 = call <vilib>:"Linear Fit.vi"("Y"=w689, "X"=w698) -> ("slope"=w679:dbl)  [unwired: 9 in, 4 out]
              n299 = call <vilib>:"Mean.vi"("X"=w689) -> ("mean"=w688:dbl)  [unwired: 1 out]
              n300 = Inverse Tangent(1:w679) -> (0:w678:dbl)
              n301 = Divide(x=w678, y=6.283185307179586) -> (x/y=w676:dbl)
              n302 = Multiply(x=w676, y=w675) -> (x*y=w674:dbl)
              n303 = case shown="2" w690 {
                tunnel: w689 -> [w709 w712 w718]
                tunnel: w679 -> [w708 w714 w720]
                tunnel: w688 -> [w707 w715 w721]
                tunnel: w683 -> [w706 w713 w719]
                tunnel: w686 -> [w705 w711 w717]
                tunnel: w674 -> [w704 w710 w716]
                frame 0, Default {
                  "slope 1" <- w708
                  "Mean Blade 1" <- w709
                  "Av Disp 1" <- w707
                  "Variance Blade 1" <- w706
                  "Av Variance 1" <- w705
                  "Angle 1" <- w704
                }
                frame 1 {
                  "Av Disp 2" <- w715
                  "Mean Blade 2" <- w712
                  "Variance Blade 2" <- w713
                  "slope 2" <- w714
                  "Av Variance 2" <- w711
                  "Angle 2" <- w710
                }
                frame 2 {
                  "Av Disp 3" <- w721
                  "Mean Blade 3" <- w718
                  "Variance Blade 3" <- w719
                  "slope 3" <- w720
                  "Av Variance 3" <- w717
                  "Angle 3" <- w716
                }
              }
            }
          }
          frame #4 {
            n304 = case shown="True" w727 {
              frame False {
              }
              frame True {
                n305 = for {
                  N: 3 -> [_]
                  tunnel: [w758] -> w749 mode=indexing
                  tunnel: [w757] -> w748 mode=indexing
                  tunnel: [w756] -> w747 mode=indexing
                  tunnel: [w755] -> w731 mode=indexing
                  i -> [w764]
                  n306 = Increment(x=w764) -> (x+1=w763:i32)
                  n307 = Format Into String(format string="Blade %d:", w763) -> (resulting string=w754:string)  [unwired: 2 in, 1 out]
                  n308 = Concatenate Strings(w754, "Angle:") -> (w755:string)
                  n309 = Concatenate Strings(w754, "Slope:") -> (w758:string)
                  n310 = Concatenate Strings(w754, "Average:X") -> (w757:string)
                  n311 = Concatenate Strings(w754, "Variance of:X") -> (w756:string)
                }
                n312 = local read "Av Variance 1"() -> (w738:dbl)
                n313 = local read "Av Variance 2"() -> (w737:dbl)
                n314 = local read "Av Variance 3"() -> (w736:dbl)
                n315 = local read "Av Disp 1"() -> (w741:dbl)
                n316 = local read "Av Disp 2"() -> (w740:dbl)
                n317 = local read "Av Disp 3"() -> (w739:dbl)
                n318 = local read "slope 1"() -> (w744:dbl)
                n319 = local read "slope 2"() -> (w743:dbl)
                n320 = local read "slope 3"() -> (w742:dbl)
                n321 = local read "Angle 3"() -> (w730:dbl)
                n322 = local read "Angle 1"() -> (w729:dbl)
                n323 = local read "Angle 2"() -> (w728:dbl)
                n324 = Build Array(w729, w728, w730, w744, w743, w742, w741, w740, w739, w738, w737, w736) -> (w735:dbl[])
                n325 = local read "Plug in values"() -> (w734:string[])
                n326 = local read "Plug in titles"() -> (w746:string[])
                n327 = for {
                  tunnel: w735 -> [w752] mode=indexing
                  tunnel: [w751] -> w733 mode=indexing
                  n328 = call "Number_2_string.vi"("number"=w752) -> ("String"=w751:string)  [unwired: 1 in]
                }
                n329 = Build Array (concatenate)(w746, w731, w749, w748, w747) -> (w745:string[])
                n330 = Build Array (concatenate)(w734, w733) -> (w732:string[])
                n331 = local write "Plug in titles"(w745) -> ()
                n332 = local write "Plug in values"(w732) -> ()
              }
            }
          }
        }
      }
      frame "Get Last Block info" {
        n333 = case shown="\"Post Process Raw Data File\"" w773 {
          tunnel: w775 -> [_ _]
          tunnel: w774 -> [_ _]
          tunnel: [w776 "Post Process"] -> w772
          tunnel: [w780 TRUE ("Processing last block?")] -> w766
          tunnel: w765 -> [w780 _]
          frame "Take New Data" {
            n334 = Select(t="Change Dem Volts", s="Change Dem Voltages?", f="Post Process") -> (s? t:f=w776:string)
          }
          frame "Post Process Raw Data File" {
          }
        }
      }
      frame "Change Dem Volts" {
        n335 = local read "All WTs"() -> (w804:dbl[][])
        n336 = for {
          tunnel: w808 -> [w836]
          tunnel: [w835] -> w807 mode=indexing
          tunnel: [w834] -> w790 mode=indexing
          tunnel: w804 -> [w832] mode=indexing
          tunnel: [w831] -> w802 mode=indexing
          tunnel: [w830] -> w784
          tunnel: w783 -> [w829]
          i -> [w837]
          n337 = Increment(x=w837) -> (x+1=w830:i32)
          n338 = Format Into String(format string=w836, w830) -> (resulting string=w834:string)  [unwired: 2 in, 1 out]
          n339 = Format Into String(format string=w829, w830) -> (resulting string=w835:string)  [unwired: 2 in, 1 out]
          n340 = Index Array(array=w832, index=0) -> (element=w831:dbl)
        }
        n341 = Build Array (concatenate)(w807, w790) -> (w806:string[])
        n342 = call "Get_Current_Scan_client.vi"("ADAM Ch Names"=w806) -> ("Numerical Values"=w805:dbl[])  [unwired: 3 out]
        n343 = Split 1D Array(array=w805, index=w784) -> (first subarray=w803:dbl[], second subarray=w801:dbl[])
        n344 = Divide(x=w803, y=w802) -> (x/y=w793:dbl[])
        n345 = In Range and Coerce(upper limit=1.05, x=w793, lower limit=0.95) -> (coerced(x)=w792:dbl[], In Range?=w791:bool[])
        n346 = Multiply(x=w792, y=w801) -> (x*y=w796:dbl[])
        n347 = In Range and Coerce(upper limit=9.9, x=w796, lower limit=0.0) -> (coerced(x)=w789:dbl[])  [unwired: 1 out]
        n348 = for {
          shift-right: [w818] -> w787
          shift-left: string[] [] -> [w819]
          shift-right: [w816] -> w788
          shift-left: dbl[] [] -> [w817]
          tunnel: w791 -> [w820] mode=indexing
          tunnel: w790 -> [w815] mode=indexing
          tunnel: w789 -> [w814] mode=indexing
          n349 = case shown="False" w820 {
            tunnel: w819 -> [w822 w828]
            tunnel: [w822 w827] -> w818
            tunnel: w817 -> [w821 w826]
            tunnel: [w821 w825] -> w816
            tunnel: w815 -> [_ w824]
            tunnel: w814 -> [_ w823]
            frame False {
            }
            frame True {
              n350 = Build Array (concatenate)(w828, w824) -> (w827:string[])
              n351 = Build Array (concatenate)(w826, w823) -> (w825:dbl[])
            }
          }
        }
        n352 = call "ASYNC_Adam_client.vi"("Values"=w788, "Channel Names"=w787) -> ()  [unwired: 2 out]
      }
      frame "Post Process" {
        n353 = Compound Arithmetic op=AND("Add Phase data to results file", w842) -> (w841:bool)
        n354 = case shown="True" w841 {
          tunnel: w840 -> [_ w852]
          tunnel: w839 -> [_ w851]
          tunnel: w838 -> [_ w850]
          frame False {
          }
          frame True {
            n355 = stacked-sequence {
              tunnel: w852 -> [w854 _]
              tunnel: w851 -> [_ w881]
              tunnel: w850 -> [_ w885]
              frame #0 {
                n356 = local read "Channel to Phase lock"() -> (w861:i32[])
                n357 = property on="Channel to Phase lock" class="LstBox (strict)"() -> ("Item Names"=w860:string[])  [unwired: 2 in, 2 out]
                n358 = local read "Plug in titles"() -> (w855:string[])
                n359 = Divide(x=360, y=w854) -> (x/y=w857:dbl)
                n360 = Increment(x=w854) -> (x+1=w853:dbl)
                n361 = for {
                  tunnel: w860 -> [w879]
                  tunnel: w861 -> [w878] mode=indexing
                  tunnel: [w877] -> w859 mode=indexing
                  n362 = Index Array(array=w879, index=w878) -> (element=w877:string)
                }
                n363 = for {
                  tunnel: w859 -> [w868] mode=indexing
                  tunnel: w857 -> [w867]
                  shift-right: [w864] -> w856
                  shift-left: w855 -> [w866]
                  tunnel: w853 -> [w862]
                  n364 = for {
                    N: w862 -> [_]
                    tunnel: w868 -> [w871]
                    tunnel: w867 -> [w875]
                    tunnel: [w873] -> w865 mode=indexing
                    tunnel: [w870] -> w863 mode=indexing
                    i -> [w876]
                    n365 = Multiply(x=w875, y=w876) -> (x*y=w869:dbl)
                    n366 = Format Into String(format string="%s:Mean:%.1f Deg:%.1f", w871, w869, w869) -> (resulting string=w873:string)  [unwired: 2 in, 1 out]
                    n367 = Format Into String(format string="%s:Variance:%.1f Deg:%.1f", w871, w869, w869) -> (resulting string=w870:string)  [unwired: 2 in, 1 out]
                  }
                  n368 = Build Array (concatenate)(w866, w865, w863) -> (w864:string[])
                }
                n369 = local write "Plug in titles"(w856) -> ()
              }
              frame #1 {
                n370 = local read "Number of Revs"() -> (w888:i32)
                n371 = Array Subset(array=w885, index (row)=1 ("index")) -> (w883:dbl[][])  [unwired: 3 in]
                n372 = Array Subset(array=w881, index (row)=1 ("index")) -> (w880:dbl[][])  [unwired: 3 in]
                n373 = local read "Plug in values"() -> (w890:string[])
                n374 = Divide(x=w880, y=w888) -> (x/y=w889:dbl[][])
                n375 = Divide(x=w883, y=w888) -> (x/y=w886:dbl[][])
                n376 = for {
                  tunnel: w889 -> [w896] mode=indexing
                  shift-right: [w894] -> w887
                  shift-left: w890 -> [w895]
                  tunnel: w886 -> [w892] mode=indexing
                  n377 = for {
                    tunnel: w896 -> [w901] mode=indexing
                    tunnel: [w902] -> w893 mode=indexing
                    tunnel: w892 -> [w900] mode=indexing
                    tunnel: [w897] -> w891 mode=indexing
                    n378 = Multiply(x=w901, y=w901) -> (x*y=w899:dbl)
                    n379 = Subtract(x=w900, y=w899) -> (x-y=w898:dbl)
                    n380 = call "Number_2_string.vi"("number"=w901) -> ("String"=w902:string)  [unwired: 1 in]
                    n381 = call "Number_2_string.vi"("number"=w898) -> ("String"=w897:string)  [unwired: 1 in]
                  }
                  n382 = Build Array (concatenate)(w895, w893, w891) -> (w894:string[])
                }
                n383 = local write "Plug in values"(w887) -> ()
              }
            }
          }
        }
        n384 = Compound Arithmetic op=AND("Save Phase averaged Profiles", w842) -> (w844:bool)
      }
      frame "Check Folder Name" {
        n385 = File/Directory Info(path="Output Directory") -> (error out=w908:errorcluster)  [unwired: 1 in, 6 out]
        n386 = Empty String/Path?(string/path="Output Directory") -> (empty?=w910:bool)
        n387 = Unbundle By Name(w908) -> ("status"=w909:bool)
        n388 = Or(x=w910, y=w909) -> (x .or. y?=w911:bool)
        n389 = case shown="True" w911 {
          tunnel: [w918 w924] -> w904
          tunnel: "Output Directory" -> [w918 w922]
          tunnel: [FALSE ("cancelled") w919] -> w906
          frame False {
          }
          frame True {
            n390 = Strip Path(path=w922) -> (stripped path=w921:path, name=w920:string)
            n391 = File Dialog(7:"Please Select a new or existing Results folder" ("prompt"), 9:w920, 11:w921) -> (1:w919:bool, 3:w924:path)  [unwired: 1 in, 5 out]
          }
        }
        n392 = local write "Output Directory"(w904) -> ()
        n393 = Not(x=w906) -> (.not. x?=w905:bool)
      }
      frame "Save Phase locked data" {
        n394 = global read "Meas_global.vi" "Raw data file"() -> (w929:path)
        n395 = stacked-sequence {
          seq-local: [_ w972 _ _] -> [_ _ _ w1029]
          seq-local: [w946 _ _ _] -> [_ _ _ w1030]
          seq-local: [_ _ w988 _] -> [_ _ _ w1028]
          seq-local: [w935 _ _ _] -> [_ _ w986 _]
          tunnel: w931 -> [_ _ _ _]
          tunnel: w929 -> [w945 _ _ w1034]
          tunnel: w927 -> [w942 _ _ _]
          tunnel: w926 -> [w941 _ _ _]
          tunnel: w925 -> [_ _ w985 _]
          frame #0 {
            w947 = "\r"
            n396 = local read "Number of Revs"() -> (w940:i32)
            n397 = Array Subset(array=w941, index (row)=1 ("index")) -> (w938:dbl[][])  [unwired: 3 in]
            n398 = Array Subset(array=w942, index (row)=1 ("index")) -> (w939:dbl[][])  [unwired: 3 in]
            n399 = for {
              tunnel: w940 -> [w955]
              tunnel: w939 -> [w954] mode=indexing
              tunnel: w938 -> [w953] mode=indexing
              tunnel: [w951] -> w937 mode=indexing
              tunnel: [w950] -> w936 mode=indexing
              n400 = Divide(x=w954, y=w955) -> (x/y=w951:dbl[])
              n401 = Divide(x=w953, y=w955) -> (x/y=w952:dbl[])
              n402 = Multiply(x=w951, y=w951) -> (x*y=w956:dbl[])
              n403 = Subtract(x=w952, y=w956) -> (x-y=w950:dbl[])
            }
            n404 = call "Read_RD_Ch_header.vi"("Raw data file"=w945) -> ("Ch string"=w949:string)  [unwired: 3 out]
            n405 = Build Array (concatenate)(w937, w936) -> (w935:dbl[][])
            n406 = Concatenate Strings(w947, "*****This is a many rows per single point file*****", w947, w949) -> (w946:string)
          }
          frame #1 {
            w958 = "\r"
            n407 = local read "Channel to Phase lock"() -> (w974:i32[])
            n408 = property on="Channel to Phase lock" class="LstBox (strict)"() -> ("Item Names"=w973:string[])  [unwired: 2 in, 2 out]
            n409 = Initialize Array("", 10) -> (w975:string[])
            n410 = call "Asterisk_header.vi"("Channel names"=w975) -> ("Header string"=w957:string)
            n411 = for {
              tunnel: w974 -> [w983] mode=indexing
              tunnel: w973 -> [w982]
              tunnel: [w981] -> w970 mode=indexing
              tunnel: ["Mean" ("format string")] -> w968 mode=indexing
              tunnel: ["Variance" ("format string")] -> w967 mode=indexing
              tunnel: [""] -> w965 mode=indexing
              n412 = Index Array(array=w982, index=w983) -> (element=w981:string)
            }
            n413 = Build Array (concatenate)("Rotor", w970, w970) -> (w964:string[])
            n414 = Build Array (concatenate)("Angle", w968, w967) -> (w963:string[])
            n415 = Build Array (concatenate)("(deg)", w965, w965) -> (w962:string[])
            n416 = Build Array(w964, w963, w962) -> (w961:string[][])
            n417 = Array To Spreadsheet String(array=w961, 3:"%s" ("format string")) -> (spreadsheet string=w959:string)  [unwired: 1 out]
            n418 = Concatenate Strings(w958, w957, w959, w958) -> (w972:string)
          }
          frame #2 {
            n419 = Array Size(array=w986) -> (size(s)=w989:i32[])
            n420 = Index Array(array=w989, index=0) -> (element=w995:i32)
            n421 = Divide(x=360, y=w985) -> (x/y=w984:dbl)
            n422 = Index Array(array=w989, index=1) -> (element=w990:i32)
            n423 = Decrement(x=w995) -> (x-1=w996:i32)
            n424 = for {
              N: w990 -> [_]
              shift-right: [w1009] -> w988
              shift-left: "" -> [w1004]
              tunnel: "Separation Character" -> [w1000]
              tunnel: w986 -> [w1007]
              tunnel: w996 -> [w1003]
              tunnel: w984 -> [w1002]
              i -> [w999]
              n425 = Index Array(array=w1007, index (col)=w999) -> (element=w1006:dbl[])  [unwired: 1 in]
              n426 = Multiply(x=w999, y=w1002) -> (x*y=w998:dbl)
              n427 = call "Number_2_string.vi"("number"=w998) -> ("String"=w997:string)  [unwired: 1 in]
              n428 = Concatenate Strings(w997, w1000) -> (w1001:string)
              n429 = for {
                shift-right: [w1017] -> w1005
                shift-left: w1001 -> [w1018]
                tunnel: w1000 -> [w1016]
                tunnel: w1006 -> [w1012] mode=indexing
                tunnel: w1003 -> [w1014]
                i -> [w1015]
                n430 = Equal?(x=w1015, y=w1014) -> (x = y?=w1013:bool)
                n431 = call "Number_2_string.vi"("precision"="precision", "number"=w1012) -> ("String"=w1011:string)
                n432 = case shown="False" w1013 {
                  tunnel: w1018 -> [w1022 w1025]
                  tunnel: w1011 -> [w1021 w1024]
                  tunnel: [w1020 w1023] -> w1017
                  tunnel: w1016 -> [w1019 _]
                  frame False {
                    n433 = Concatenate Strings(w1022, w1021, w1019) -> (w1020:string)
                  }
                  frame True {
                    n434 = Concatenate Strings(w1025, w1024) -> (w1023:string)
                  }
                }
              }
              n435 = Concatenate Strings(w1004, w1005, "\r") -> (w1009:string)
            }
          }
          frame #3 {
            w1026 = FALSE  # append to file? (new file:F)
            n436 = Strip Path(path=w1034) -> (name=w1032:string)  [unwired: 1 out]
            n437 = local read "Output Directory"() -> (w1033:path)
            n438 = Build Path(base path=w1033, name or relative path=w1032) -> (appended path=w1031:path)
            n439 = Concatenate Strings(w1030, w1029, w1028) -> (w1027:string)
            n440 = call "Write_File_Simple.vi"("append to file? (new file:F)"=w1026, "character string"=w1027, "file path"=w1031) -> ()  [unwired: 2 out]
          }
        }
      }
    }
  }
